vi "do_move.vi"(5 "Trio handle":refnum<k7>, 7 "Absolute":bool, 8 "error in":errorcluster, 9 "Axis positions":dbl[](array[numeric]), 10 "Axis enable":bool[](array[boolean]), 11 "Newmark handle":refnum<visa-resource-name>) -> (0 "error out":errorcluster)   [LabVIEW 2024]
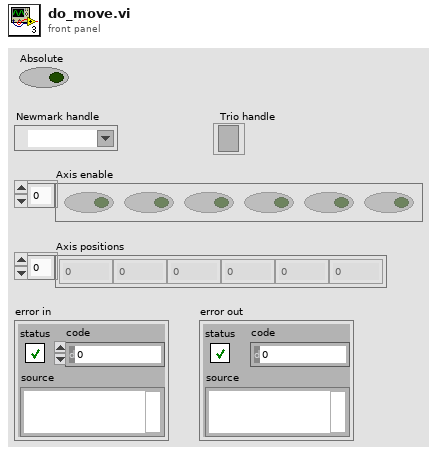
[diagram p1: front panel]
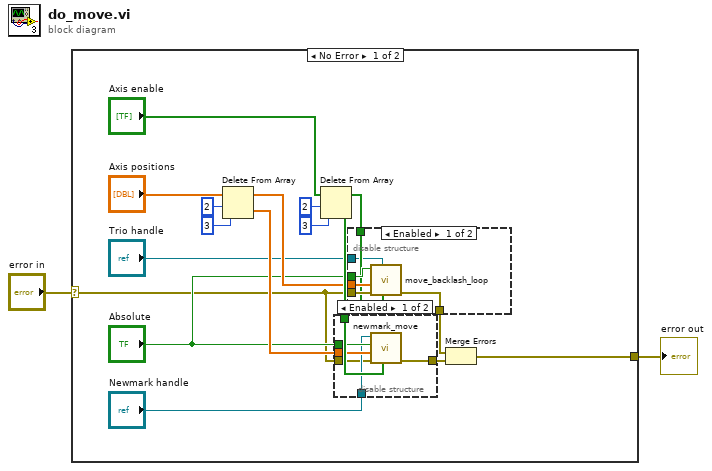
[diagram p0: block diagram]
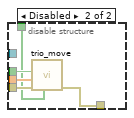
[diagram p3: hidden frame]
diagram:
  n1 = case shown="No Error" "error in" {
    selector: "error in" -> [w5 w37]
    tunnel: [w4 w37] -> w2
    frame No Error {
      n2 = Delete From Array(array="Axis positions", length=2, index=3) -> (deleted portion=w15:dbl[], array with subset deleted=w14:dbl[])
      n3 = Delete From Array(array="Axis enable", length=2, index=3) -> (deleted portion=w19:bool[], array with subset deleted=w18:bool[])
      n4 = disable-structure shown="Enabled" {
        disable-tunnel: w19 -> [w25 _]
        disable-tunnel: w15 -> [w24 _]
        disable-tunnel: [w23 _] -> w11
        disable-tunnel: "Absolute" -> [w22 _]
        disable-tunnel: "Newmark handle" -> [w21 _]
        disable-tunnel: w5 -> [w20 _]
        frame Enabled {
          n5 = call "newmark_move.vi"("Axis enable"=w25, "error in"=w20, "Axis positions"=w24, "Absolute"=w22, "VISA Refnum in"=w21) -> ("error out"=w23:errorcluster)  [unwired: 4 in, 2 out]
        }
        frame Disabled {
        }
      }
      n6 = disable-structure shown="Enabled" {
        disable-tunnel: "Absolute" -> [w31 w36]
        disable-tunnel: w5 -> [w30 w35]
        disable-tunnel: [w29 w34] -> w10
        disable-tunnel: w14 -> [w28 w33]
        disable-tunnel: w18 -> [w27 w32]
        disable-tunnel: "Trio handle" -> [w26 _]
        frame Enabled {
          n7 = call "move_backlash_loop.vi"("Axis enable"=w27, "Trio handle"=w26, "error in"=w30, "Axis positions"=w28, "Absolute"=w31) -> ("error out"=w29:errorcluster)  [unwired: 5 in, 1 out]
        }
        frame Disabled {
          n8 = call "trio_move.vi"("Axis enable"=w32, "error in"=w35, "Axis positions"=w33, "Absolute"=w36) -> ("error out"=w34:errorcluster)  [unwired: 6 in, 1 out]
        }
      }
      n9 = Merge Errors(w10, w11) -> (w4:errorcluster)
    }
    frame Error {
    }
  }
  "error out" <- w2
